vi "Write Tiff File.vi"(4 "Tags":T4(array[cluster]), 5 "Named Tags":T6(array[cluster]), 6 "Settings":T5={"zlib compression level"=-1, "Max Strip bytes"=8192, "JPEG Quality (85)"=85}, 7 "Pages":cluster{"Image Data":variant, "Details":T7}[](array[cluster]) {"Details"."PhotometricInterpretation" items=["PHOTOMETRIC_MINISWHITE"=0, "PHOTOMETRIC_MINISBLACK"=1, "PHOTOMETRIC_RGB"=2, "PHOTOMETRIC_PALETTE"=3, "PHOTOMETRIC_MASK"=4, "PHOTOMETRIC_SEPARATED"=5, "PHOTOMETRIC_YCBCR"=6, "PHOTOMETRIC_CIELAB"=8, "PHOTOMETRIC_ICCLAB"=9, "PHOTOMETRIC_ITULAB"=10, "PHOTOMETRIC_LOGL"=32844, "PHOTOMETRIC_LOGLUV"=32845, "CFA"=32803, "LinearRaw"=34892, "DEPTH"=51177]}, 8 "error in (no error)":errorcluster, 10 "operation (replace)":T1(ring)=enum."replace or create", 11 "Path":path) -> (0 "error out":errorcluster, 3 "path":path)   [LabVIEW 2020, in "LV Tiff.lvlib" / "TIFF Writer.lvclass"]
uses:
  TIFF Writer.lvclass
  _Helpers/Tiff Page Details.ctl
  _Helpers/Page Writer Settings.ctl
  _Helpers/Tiff Data Type.ctl
  TIFF Writer.lvclass/TIFF Writer.ctl
  LV Tiff.lvlib
  _Helpers/Tiff Tags.ctl
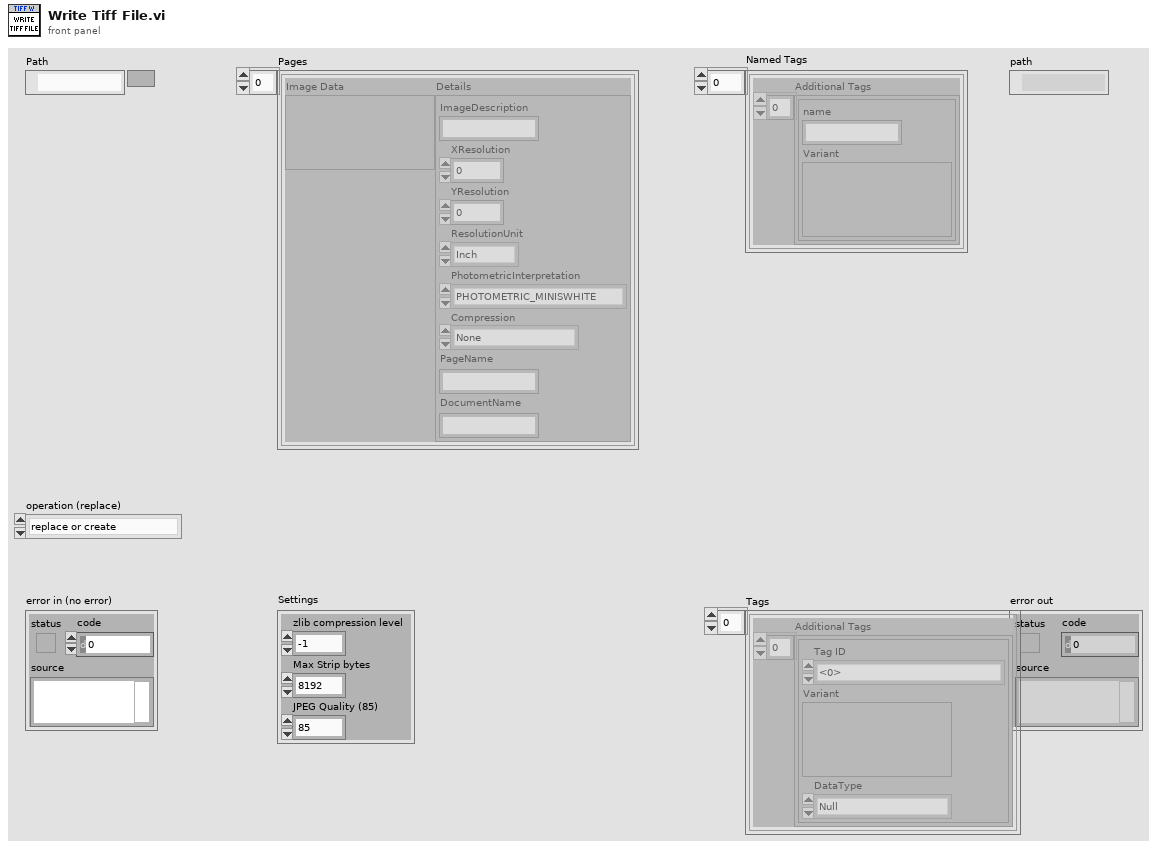
[diagram p1: front panel]
types:
  T1 = enum16{"open", "replace", "create", "open or create", "replace or create", "replace or create with confirmation"}
  T2 = typedef "LV Tiff.lvlib/Tiff Tags.ctl" = u16
  T3 = typedef "LV Tiff.lvlib/Tiff Data Type.ctl" = enum16{"Null", "BYTE", "ASCII", "SHORT", "LONG", "RATIONAL", "SBYTE", "UNDEFINE", "SSHORT", "SLONG", "SRATIONAL", "FLOAT", "DOUBLE"}
  T4 = cluster{"Additional Tags":cluster{"Tag ID":T2, "Variant":variant, "DataType":T3}[]}[]
  T5 = typedef "LV Tiff.lvlib/Page Writer Settings.ctl" = cluster{"zlib compression level":i32, "Max Strip bytes":u32, "JPEG Quality (85)":i32}
  T6 = cluster{"Additional Tags":cluster{"name":string, "Variant":variant}[]}[]
  T7 = typedef "LV Tiff.lvlib/Tiff Page Details.ctl" = cluster{"ImageDescription":string, "XResolution":dbl, "YResolution":dbl, "ResolutionUnit":enum16{"None", "Inch", "Centimeter"}, "PhotometricInterpretation":u16, "Compression":enum16{"None", "Deflate", "JPEG"}, "PageName":string, "DocumentName":string}
  T8 = cluster{"Additional Tags":cluster{"name":string, "Variant":variant}[]}
  T9 = cluster{"Additional Tags":cluster{"Tag ID":T2, "Variant":variant, "DataType":T3}[]}
  T10 = cluster{"Tag ID":T2, "Variant":variant, "DataType":T3}[]
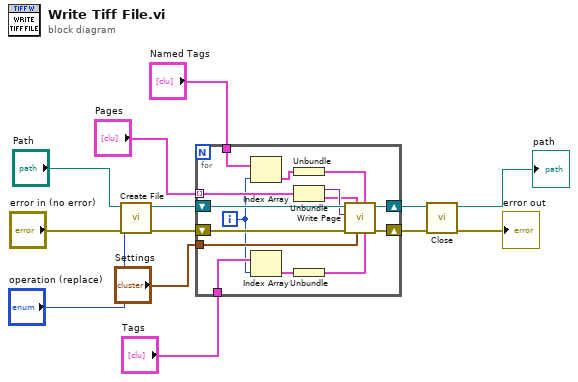
[diagram p0: block diagram]
diagram:
  n1 = call "Create File.vi"("error in (no error)"="error in (no error)", "operation (replace)"="operation (replace)", "Path"="Path") -> ("error out"=w10:errorcluster, "TIFF Writer out"=w12:refnum<class "TIFF Writer.lvclass">)  [unwired: 7 in]
  n2 = for {
    shift-right: [w27] -> w11
    shift-left: w12 -> [w28]
    shift-right: [w25] -> w9
    shift-left: w10 -> [w26]
    tunnel: "Named Tags" -> [w24]
    tunnel: "Pages" -> [w23] mode=indexing
    tunnel: "Settings" -> [w18]
    tunnel: "Tags" -> [w17]
    i -> [w14]
    n3 = Index Array(array=w24, index=w14) -> (element=w22:T8)
    n4 = Index Array(array=w17, index=w14) -> (element=w15:T9)
    n5 = Unbundle(w22) -> ("Additional Tags"=w21:cluster{"name":string, "Variant":variant}[])
    n6 = Unbundle(w23) -> ("Image Data"=w20:variant, "Details"=w19:T7)
    n7 = Unbundle(w15) -> ("Additional Tags"=w16:T10)
    n8 = call "Write Page.vi"("Additional Tags"=w16, "Additional Named Tags"=w21, "Settings"=w18, "Details"=w19, "error in (no error)"=w26, "Image"=w20, "TIFF Writer in"=w28) -> ("error out"=w25:errorcluster, "TIFF Writer out"=w27:refnum<class "TIFF Writer.lvclass">)  [unwired: 3 in]
  }
  n9 = call "Close.vi"("error in (no error)"=w9, "TIFF Writer in"=w11) -> ("error out"=→"error out":errorcluster, "path"=→"path":path)  [unwired: 8 in]
